vi "Write rendezvous.vi"(8 "error in (no error)":errorcluster, 10 "rendezvous":T1, 11 "UV-VIS_AVANTES in":refnum<class "UV-VIS_AVANTES.lvclass">) -> (0 "error out":errorcluster, 3 "UV-VIS_AVANTES out":refnum<class "UV-VIS_AVANTES.lvclass">)   [LabVIEW 2020, in "UV-VIS_AVANTES.lvclass"]
uses:
  UV-VIS_AVANTES.lvclass
  UV-VIS_AVANTES.lvclass/UV-VIS_AVANTES.ctl
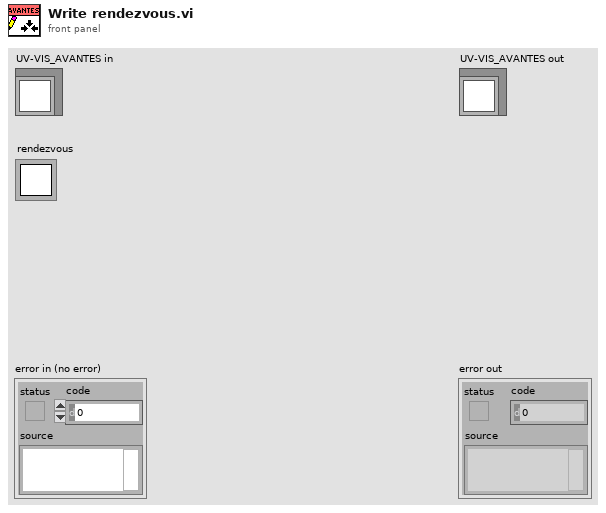
[diagram p1: front panel]
types:
  T1 = typedef "Rendezvous RefNum" = refnum<k1>
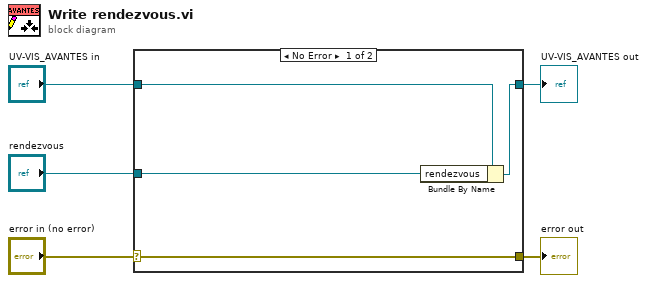
[diagram p0: block diagram]
diagram:
  n1 = case shown="No Error" "error in (no error)" {
    selector: "error in (no error)" -> [w9 w10]
    tunnel: [w9 w10] -> w4
    tunnel: [w7 w11] -> w2
    tunnel: "UV-VIS_AVANTES in" -> [w8 w11]
    tunnel: "rendezvous" -> [w6 _]
    frame No Error {
      n2 = Bundle By Name(cluster=w8, "rendezvous"=w6) -> (w7:refnum<class "UV-VIS_AVANTES.lvclass">)
    }
    frame Error {
    }
  }
  "error out" <- w4
  "UV-VIS_AVANTES out" <- w2
